vi "Init Channel Read Array.vi"(8 "error in":errorcluster, 11 "Init Channels In":refnum<class "Init Channels.lvclass">) -> (0 "error out":errorcluster, 1 "Changed or First Call?":bool, 2 "Init Channels ACT":bool[](array[boolean]), 3 "Init Channels Out":refnum<class "Init Channels.lvclass">)   [LabVIEW 2023, in "Init Channels.lvclass"]
uses:
  Init Channels.lvclass
  0965f846-d7e0-43d3-b41b-98988485e72c.vi
  <vilib>/ADAS Replay HIL/Channels/Tag Wrapper/Tag Wrapper.lvlib
  <vilib>/ADAS Replay HIL/Channels/Tag Wrapper/Polymorphic/Read Channel (Boolean).vi
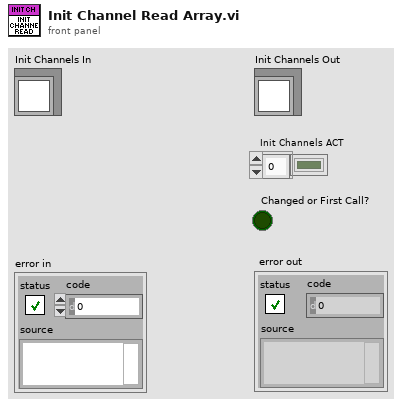
[diagram p1: front panel]
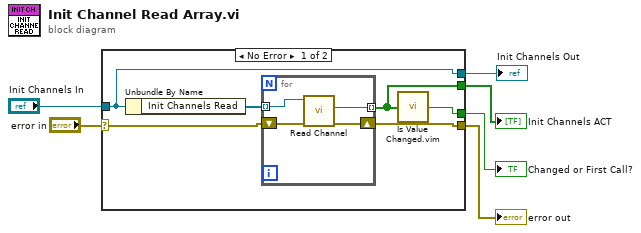
[diagram p0: block diagram]
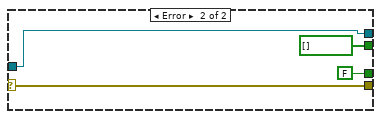
[diagram p2: hidden frame]
diagram:
  n1 = case shown="No Error" "error in" {
    selector: "error in" -> [w12 w20]
    tunnel: [w11 w20] -> w5
    tunnel: [w7 w19] -> w1
    tunnel: "Init Channels In" -> [w7 w19]
    tunnel: [w10 bool[] []] -> w3
    tunnel: [w9 FALSE ("changed or first call?")] -> w4
    frame No Error {
      n2 = Unbundle By Name(w7) -> ("Init Channels Read"=w8:refnum<k21>[])
      n3 = for {
        tunnel: [w14] -> w10 mode=indexing
        shift-right: [w15] -> w11
        shift-left: w12 -> [w16]
        tunnel: w8 -> [w13] mode=indexing
        n4 = call-poly <vilib>:"Read Channel.vi"("error in"=w16, "ADAS HIL Channel in"=w13) -> ("error out"=w15:errorcluster, "Value out"=w14:bool)  [unwired: 6 in, 2 out]
      }
      n5 = call "Is Value Changed.vim"("value"=w10) -> ("changed or first call?"=w9:bool)
    }
    frame Error {
    }
  }
  "error out" <- w5
  "Changed or First Call?" <- w4
  "Init Channels ACT" <- w3
  "Init Channels Out" <- w1
